vi "CRYPlot Data by Legend.vi"(4 "Flattened Scale Property":string, 5 "Frequency Symbols":i32[](array[numeric]), 6 "Flattened Plot Property":string, 7 "pGraph VI":refnum<vi>, 8 "Legend Symbols":i32[](array[numeric]), 9 "Result Rows":i32[](array[numeric]), 10 "Value Rows":i32[](array[numeric]), 11 "Rows":i32[](array[numeric])) -> ()   [LabVIEW 2013]
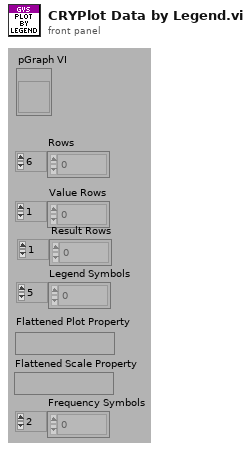
[diagram p1: front panel]
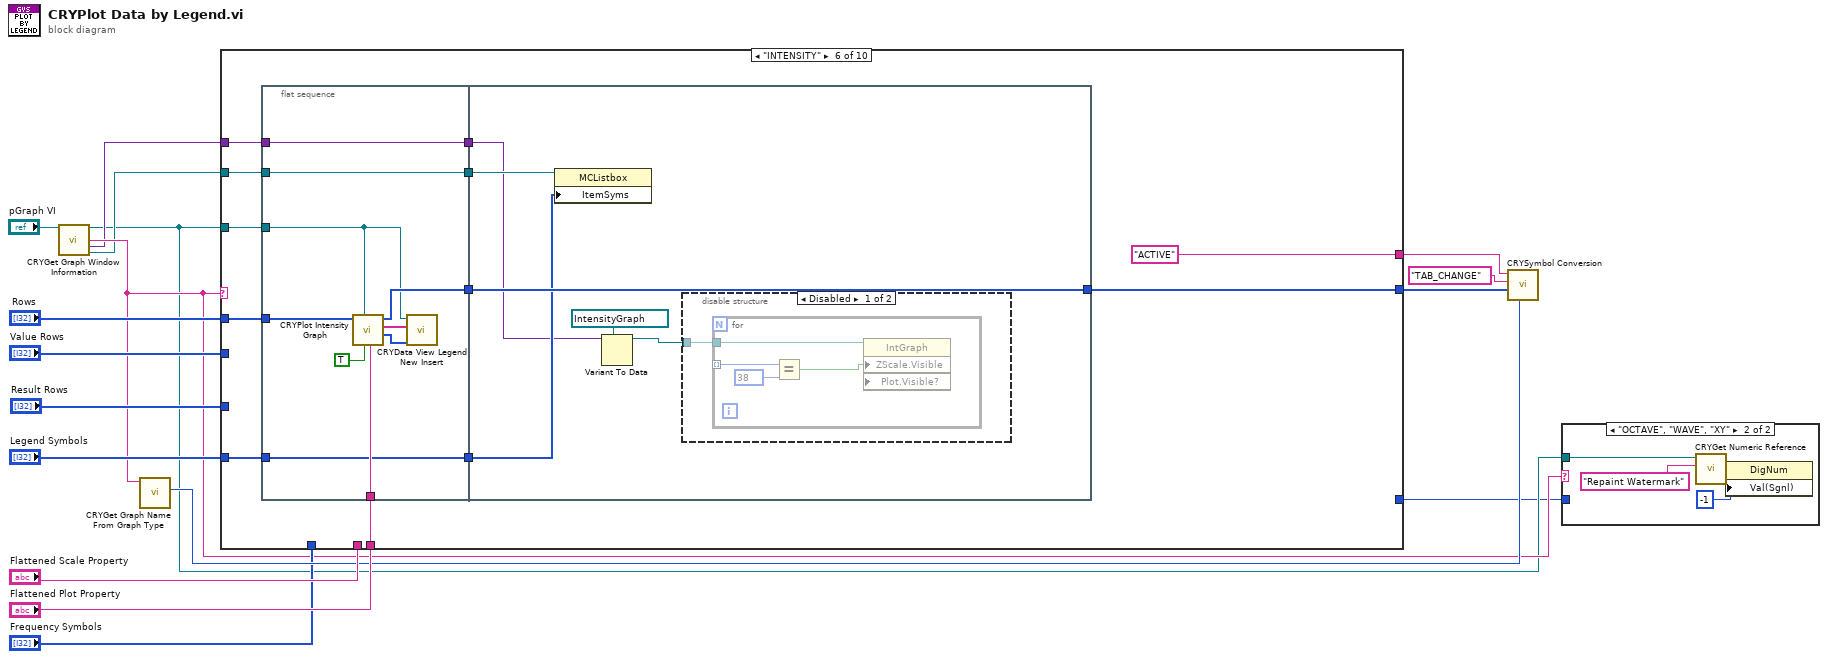
[diagram p0: block diagram]
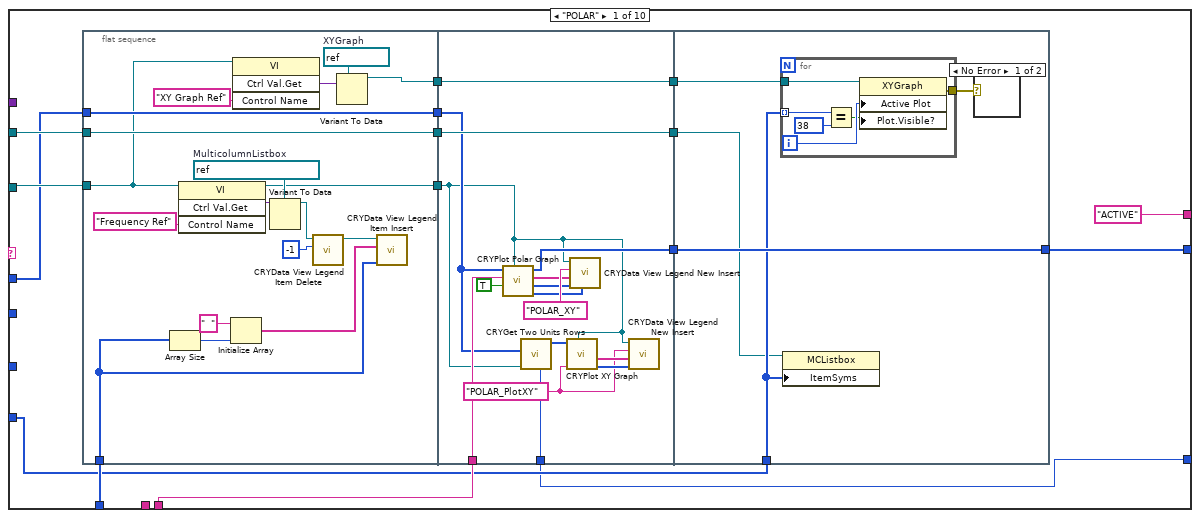
[diagram p3: hidden frame]
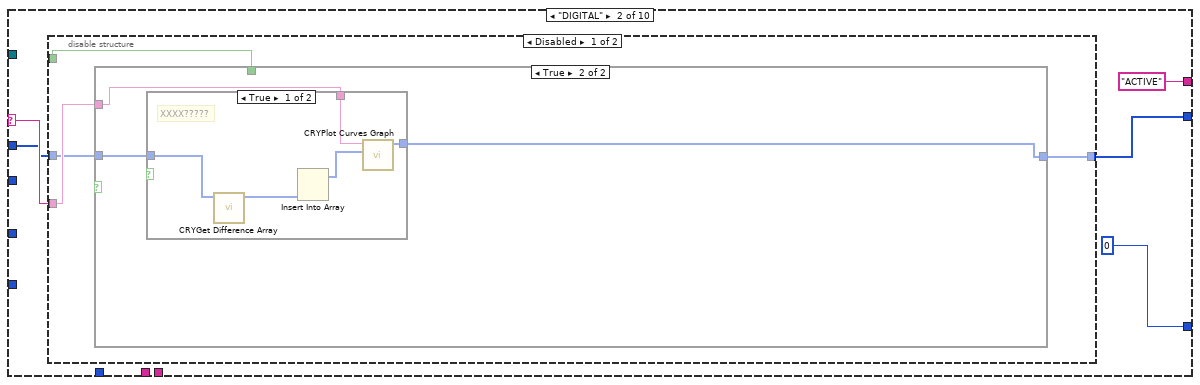
[diagram p5: hidden frame]
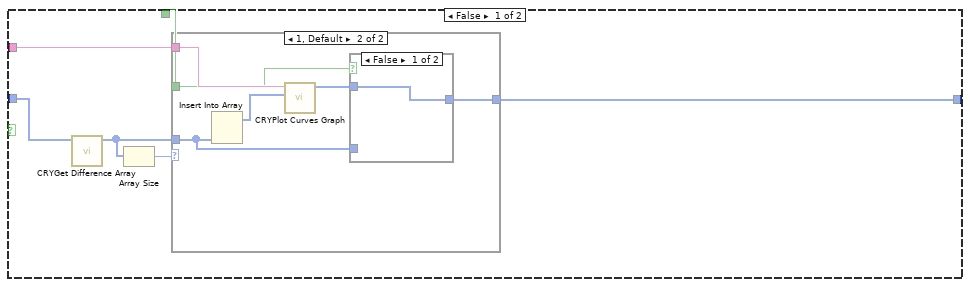
[diagram p6: hidden frame]
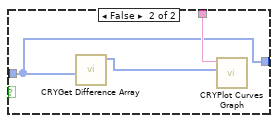
[diagram p9: hidden frame]
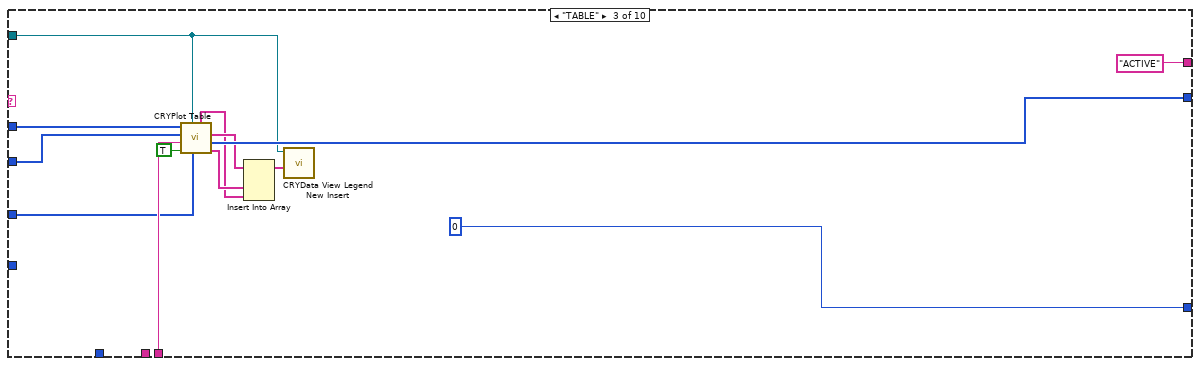
[diagram p11: hidden frame]
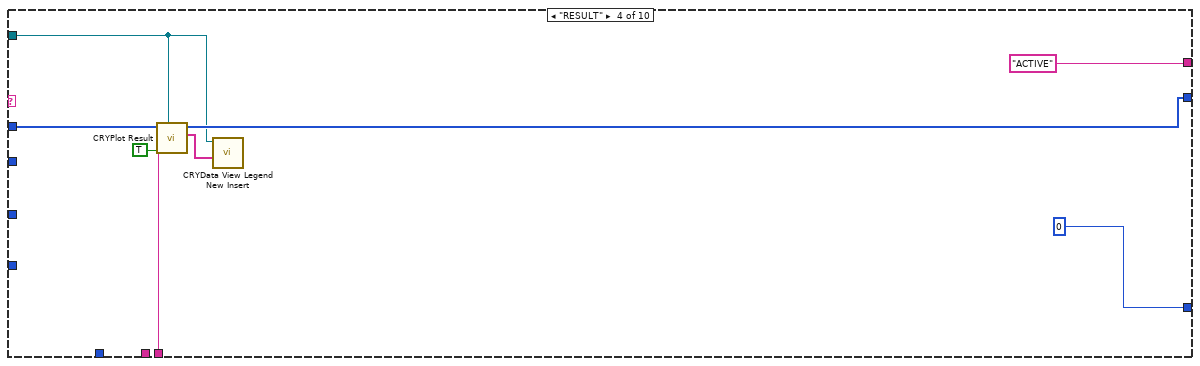
[diagram p12: hidden frame]
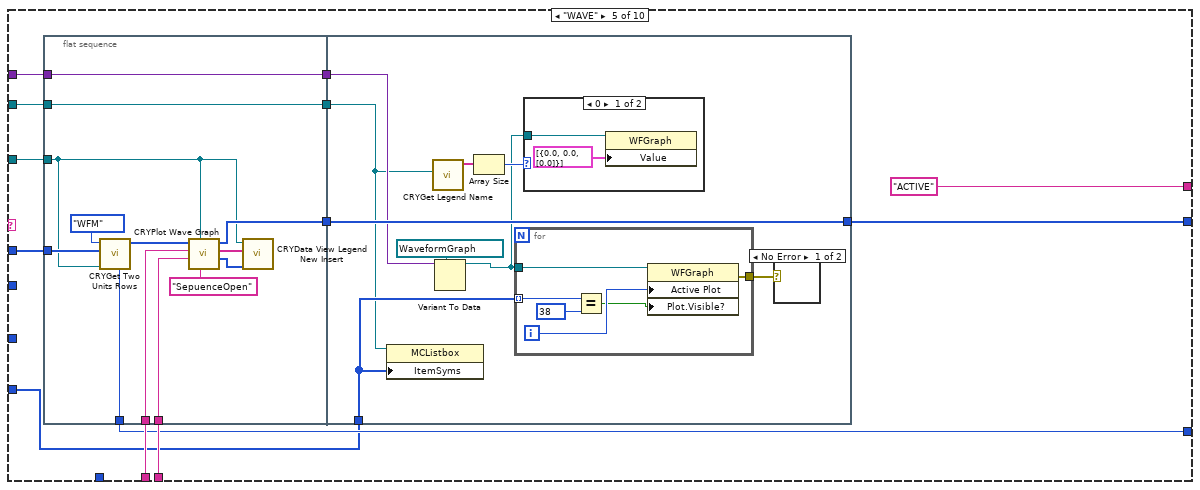
[diagram p13: hidden frame]
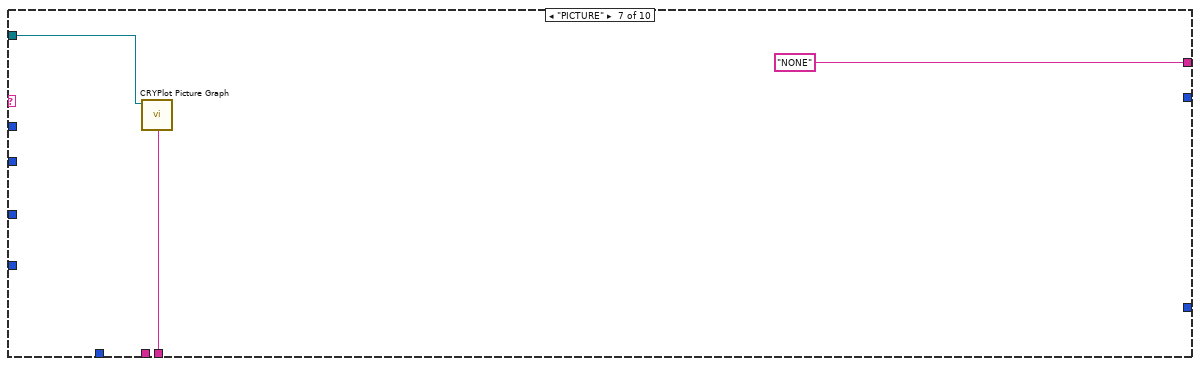
[diagram p17: hidden frame]
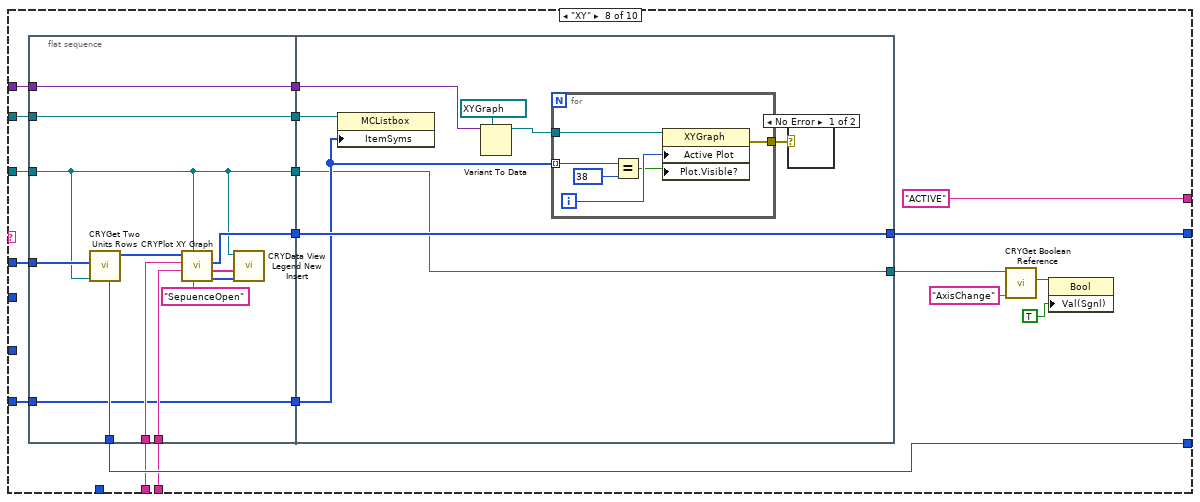
[diagram p18: hidden frame]
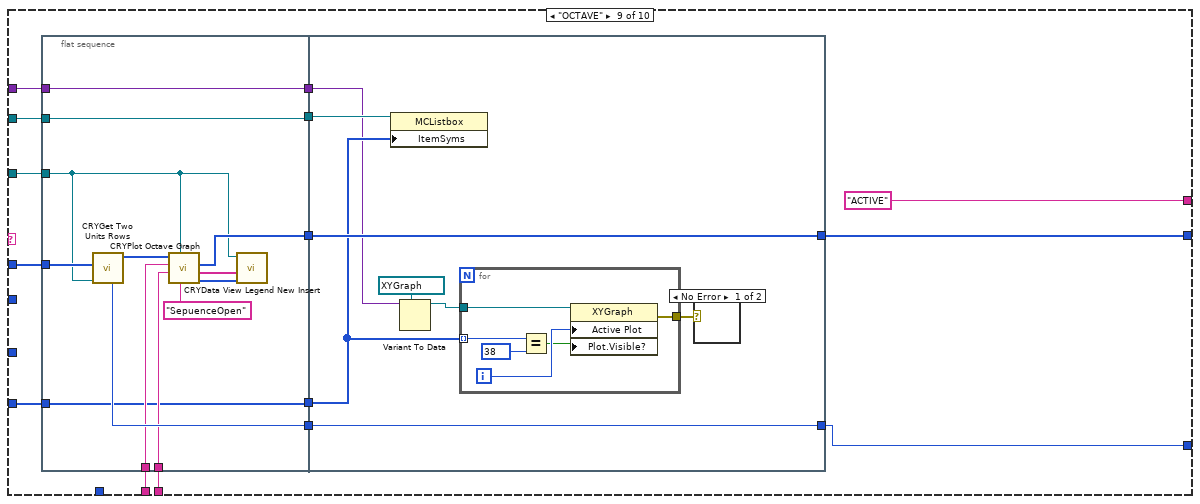
[diagram p20: hidden frame]
diagram:
  n1 = call "CRYGet Graph Window Information.vi"("pGraph VI In"="pGraph VI") -> ("pGraph VI Out"=w5:refnum<vi>, "Graph Type Out"=w9:string, "Graph Control Ref Out"=w8:variant, "Legend Ref Out"=w7:refnum<vi>)  [unwired: 4 in, 7 out]
  n2 = call "CRYGet Graph Name From Graph Type.vi"("Graph Type"=w9) -> ("Type"=w11:enum16{"Curves", "Values", "Results", "WFM"})  [unwired: 10 out]
  n3 = case shown="\"INTENSITY\"" w9 {
    selector: w9 -> [_ w83 _ _ _ _ _ _ _ _]
    tunnel: "Rows" -> [w20 w82 w121 w134 w144 w187 _ w232 w274 _]
    tunnel: [w26 0 ("Two Units") 0 ("Two Units") 0 ("Two Units") w143 _ _ w231 w273 0 ("Two Units")] -> w4
    tunnel: "Legend Symbols" -> [w27 _ _ _ w135 w185 _ w220 w266 _]
    tunnel: "Value Rows" -> [_ _ w120 _ _ _ _ _ _ _]
    tunnel: "Flattened Scale Property" -> [_ _ _ _ w146 _ _ w230 w272 _]
    tunnel: "Flattened Plot Property" -> [w31 _ w125 w132 w147 w189 w213 w229 w271 _]
    tunnel: "Result Rows" -> [_ _ w123 _ _ _ _ _ _ _]
    tunnel: [w30 w80 w122 w130 w145 w188 _ w228 w270 i32[] [] ("All Rows Out")] -> w2
    tunnel: ["ACTIVE" ("sActin") "ACTIVE" ("sActin") "ACTIVE" ("sActin") "ACTIVE" ("sActin") "ACTIVE" ("sActin") "ACTIVE" ("sActin") "NONE" ("sActin") "ACTIVE" ("sActin") "ACTIVE" ("sActin") "ACTIVE" ("sActin")] -> w1
    tunnel: w5 -> [w32 _ w114 w127 w141 w184 w211 w219 w260 _]
    tunnel: "Frequency Symbols" -> [w29 _ _ _ _ _ _ _ _ _]
    tunnel: w8 -> [_ _ _ _ w140 w178 _ w221 w267 _]
    tunnel: w7 -> [w24 _ _ _ w139 w180 _ w223 w268 _]
    frame "POLAR" {
      n4 = flat-sequence {
        tunnel: w32 -> [w40]
        tunnel: w29 -> [w34]
        tunnel: [w37] -> w25
        tunnel: w24 -> [w46]
        tunnel: [w46] -> w22
        tunnel: [w45] -> w21
        tunnel: w20 -> [w45]
        tunnel: [w41] -> w18
        tunnel: w31 -> [w63]
        tunnel: [w62] -> w28
        tunnel: [w58] -> w26
        tunnel: w25 -> [w52]
        tunnel: [w56] -> w23
        tunnel: w22 -> [w56]
        tunnel: w21 -> [w55]
        tunnel: [w54] -> w19
        tunnel: w18 -> [w54]
        tunnel: [w72] -> w30
        tunnel: w28 -> [w72]
        tunnel: w27 -> [w71]
        tunnel: w23 -> [w70]
        tunnel: w19 -> [w68]
        frame #0 {
          w42 = refnum<vi> refnum  # XYGraph
          w49 = refnum<vi> refnum  # MulticolumnListbox
          n5 = Array Size(array=w34) -> (size(s)=w47:i32)
          n6 = invoke class="VI" method="Ctrl Val.Get"(reference=w40, "Control Name"="Frequency Ref") -> (reference out=w37:refnum<vi>, "Get Control Value Variant"=w51:variant)  [unwired: 2 in, 2 out]
          n7 = Initialize Array("  ", w47) -> (w35:string[])
          n8 = invoke class="VI" method="Ctrl Val.Get"(reference=w40, "Control Name"="XY Graph Ref") -> ("Get Control Value Variant"=w43:variant)  [unwired: 2 in, 3 out]
          n9 = Variant To Data(type=w49, Variant=w51) -> (data=w36:refnum<vi>)  [unwired: 1 in, 1 out]
          n10 = call "CRYData View Legend Item Delete.vi"("RowNumber"=-1, "Legend MultiListbox In"=w36) -> ("Legend MultiListbox Out"=w39:refnum<vi>)  [unwired: 9 out]
          n11 = Variant To Data(type=w42, Variant=w43) -> (data=w41:refnum<vi>)  [unwired: 1 in, 1 out]
          n12 = call "CRYData View Legend Item Insert.vi"("Item Symbols"=w34, "ItemName Array"=w35, "Legend MultiListbox"=w39) -> ()  [unwired: 1 in, 8 out]
        }
        frame #1 {
          w53 = "POLAR_PlotXY" ("sOption")
          n13 = call "CRYPlot Polar Graph.vi"("pGraph VI In"=w52, "GraphSet"=TRUE, "Flattened Polar Property"=w63, "Selected Rows In"=w55) -> ("ItemSyms"=w57:i32[], "Freq Color"=w64:u32[], "Freq Name"=w65:string[], "Selected Row Out"=w62:i32[])  [unwired: 2 in, 2 out]
          n14 = call "CRYGet Two Units Rows.vi"("pGraph VI In"=w52, "Old Rows In"=w55) -> ("All Rows Out"=w59:i32[], "Two Units"=w58:i32)  [unwired: 3 in, 5 out]
          n15 = call "CRYPlot XY Graph.vi"("pGraph VI In"=w52, "sType"=w53, "Selected Rows In"=w59) -> ("Color Info"=w61:u32[], "Curve Name"=w60:string[])  [unwired: 3 in, 4 out]
          n16 = call "CRYData View Legend New Insert.vi"("Item Symbols"=w57, "Color Array"=w64, "ItemName Array"=w65, "sOption"="POLAR_XY", "pGraph VI In"=w52) -> ()  [unwired: 7 out]
          n17 = call "CRYData View Legend New Insert.vi"("Color Array"=w61, "ItemName Array"=w60, "sOption"=w53, "pGraph VI In"=w52) -> ()  [unwired: 1 in, 7 out]
        }
        frame #2 {
          n18 = for {
            tunnel: w71 -> [w77] mode=indexing
            tunnel: w68 -> [w74]
            tunnel: [w73] -> w69
            i -> [w76]
            n19 = Equal?(x=w77, y=38) -> (x = y?=w75:bool)
            n20 = property class="XYGraph"(reference=w74, "Active Plot"=w76, "Plot.Visible?"=w75) -> (error out=w73:errorcluster)  [unwired: 1 in, 1 out]
          }
          n21 = property on="Property Node" class="MCListbox"(reference=w70, "ItemSyms"=w71) -> ()  [unwired: 1 in, 2 out]
          n22 = case shown="No Error" w69 {
            frame No Error {
            }
            frame Error {
            }
          }
        }
      }
    }
    frame "DIGITAL" {
      n23 = disable-structure shown="Disabled" {
        disable-tunnel: w83 -> [w87 _]
        disable-tunnel: w82 -> [w86 _]
        disable-tunnel: _ -> [w85 _]
        disable-tunnel: [w84 _] -> w80
        frame Disabled {
          n24 = case shown="True" {
            selector: _ -> [_ _]
            tunnel: w87 -> [w91 w105]
            tunnel: w86 -> [w90 w104]
            tunnel: w85 -> [w89 _]
            tunnel: [w88 w103] -> w84
            frame False {
              n25 = call "CRYGet Difference Array.vi"("Array 1"=w90) -> ("Diff Out"=w93:i32[])  [unwired: 4 in, 6 out]
              n26 = Array Size(array=w93) -> (size(s)=w92:i32)
              n27 = case shown="1, Default" w92 {
                tunnel: w91 -> [_ w99]
                tunnel: w93 -> [w94 w97]
                tunnel: w89 -> [_ w96]
                tunnel: [w94 w95] -> w88
                frame 0 {
                }
                frame 1, Default {
                  n28 = Insert Into Array(new element=w97) -> (w100:i32[])  [unwired: 2 in]
                  n29 = call "CRYPlot Curves Graph.vi"("Rows In"=w100, "Graph Type"=w99) -> ("All Rows Out"=w98:i32[])  [unwired: 8 in, 1 out]
                  n30 = case shown="False" w96 {
                    tunnel: w98 -> [w101 _]
                    tunnel: w97 -> [_ w102]
                    tunnel: [w101 w102] -> w95
                    frame False {
                    }
                    frame True {
                    }
                  }
                }
              }
            }
            frame True {
              n31 = case shown="True" {
                selector: _ -> [_ _]
                tunnel: w105 -> [w109 w113]
                tunnel: w104 -> [w108 w111]
                tunnel: [w106 w111] -> w103
                frame True {
                  # "XXXX?????"
                  n32 = call "CRYGet Difference Array.vi"("Array 1"=w108) -> ("Diff Out"=w110:i32[])  [unwired: 4 in, 6 out]
                  n33 = Insert Into Array(new element=w110) -> (w107:i32[])  [unwired: 2 in]
                  n34 = call "CRYPlot Curves Graph.vi"("Rows In"=w107, "Graph Type"=w109) -> ("All Rows Out"=w106:i32[])  [unwired: 8 in, 1 out]
                }
                frame False {
                  n35 = call "CRYGet Difference Array.vi"("Array 2"=w111) -> ("Diff Out"=w112:i32[])  [unwired: 4 in, 6 out]
                  n36 = call "CRYPlot Curves Graph.vi"("Rows In"=w112, "Graph Type"=w113) -> ()  [unwired: 8 in, 2 out]
                }
              }
            }
          }
        }
        frame Enabled {
        }
      }
    }
    frame "TABLE" {
      n37 = call "CRYPlot Table.vi"("Result Rows In"=w123, "pGraph VI In"=w114, "Graph Set?"=TRUE, "Flattened Property"=w125, "Value Rows In"=w120, "Curve Rows In"=w121) -> ("Value Name"=w117:string[], "Value Rows Out"=w122:i32[], "Curve Name"=w118:string[], "Result Name"=w116:string[])  [unwired: 2 out]
      n38 = Insert Into Array(array=w118, new element #1=w117, new element #2=w116) -> (w119:string[])  [unwired: 1 in]
      n39 = call "CRYData View Legend New Insert.vi"("ItemName Array"=w119, "pGraph VI In"=w114) -> ()  [unwired: 3 in, 7 out]
    }
    frame "RESULT" {
      n40 = call "CRYPlot Result.vi"("pGraph VI In"=w127, "Graph Set?"=TRUE, "Flattened Property"=w132, "Old Rows In"=w134) -> ("Curve Name"=w129:string[], "Selected Rows Out"=w130:i32[])  [unwired: 2 in, 4 out]
      n41 = call "CRYData View Legend New Insert.vi"("ItemName Array"=w129, "pGraph VI In"=w127) -> ()  [unwired: 3 in, 7 out]
    }
    frame "WAVE" {
      n42 = flat-sequence {
        tunnel: w147 -> [w158]
        tunnel: w146 -> [w157]
        tunnel: w144 -> [w155]
        tunnel: [w154] -> w143
        tunnel: w141 -> [w148]
        tunnel: w140 -> [w150]
        tunnel: w139 -> [w149]
        tunnel: [w156] -> w138
        tunnel: [w150] -> w137
        tunnel: [w149] -> w136
        tunnel: [w169] -> w145
        tunnel: w138 -> [w169]
        tunnel: w137 -> [w165]
        tunnel: w136 -> [w161]
        tunnel: w135 -> [w166]
        frame #0 {
          n43 = call "CRYGet Two Units Rows.vi"("pGraph VI In"=w148, "Old Rows In"=w155, "Type"=enum16{"Curves", "Values", "Results", "WFM"}."WFM") -> ("All Rows Out"=w153:i32[], "Two Units"=w154:i32)  [unwired: 2 in, 5 out]
          n44 = call "CRYPlot Wave Graph.vi"("sOption"="SepuenceOpen", "pGraph VI In"=w148, "Flattened Plot Property"=w158, "Flattened Scale Property"=w157, "Selected Rows In"=w153) -> ("Color Info"=w159:u32[], "Curve Name"=w160:string[], "Selected Rows Out"=w156:i32[])  [unwired: 1 in, 3 out]
          n45 = call "CRYData View Legend New Insert.vi"("Color Array"=w159, "ItemName Array"=w160, "pGraph VI In"=w148) -> ()  [unwired: 2 in, 7 out]
        }
        frame #1 {
          n46 = property on="Property Node" class="MCListbox"(reference=w161, "ItemSyms"=w166) -> ()  [unwired: 1 in, 2 out]
          n47 = call "CRYGet Legend Name.vi"("MCListbox Refnum"=w161) -> ("Names Out"=w163:string[])  [unwired: 2 in, 8 out]
          n48 = Variant To Data(type=refnum<vi> refnum ("WaveGraph Ref"), Variant=w165) -> (data=w162:refnum<vi>)  [unwired: 1 in, 1 out]
          n49 = Array Size(array=w163) -> (size(s)=w164:i32)
          n50 = for {
            tunnel: w166 -> [w176] mode=indexing
            tunnel: w162 -> [w173]
            tunnel: [w172] -> w167
            i -> [w175]
            n51 = Equal?(x=w176, y=38) -> (x = y?=w174:bool)
            n52 = property class="WFGraph"(reference=w173, "Active Plot"=w175, "Plot.Visible?"=w174) -> (error out=w172:errorcluster)  [unwired: 1 in, 1 out]
          }
          n53 = case shown="0" w164 {
            tunnel: w162 -> [w171 _]
            frame 0 {
              n54 = property class="WFGraph"(reference=w171, "Value"=cluster{"xo":dbl, "dx":dbl, dbl[]}[] [{"xo"=0.0, "dx"=0.0, [0.0]}] ("appended array")) -> ()  [unwired: 1 in, 2 out]
            }
            frame 1, Default {
            }
          }
          n55 = case shown="No Error" w167 {
            frame No Error {
            }
            frame Error {
            }
          }
        }
      }
    }
    frame "INTENSITY" {
      n56 = flat-sequence {
        tunnel: w189 -> [w197]
        tunnel: w187 -> [w194]
        tunnel: w185 -> [w193]
        tunnel: w184 -> [w190]
        tunnel: [w195] -> w183
        tunnel: [w193] -> w182
        tunnel: [w192] -> w181
        tunnel: w180 -> [w192]
        tunnel: [w191] -> w179
        tunnel: w178 -> [w191]
        tunnel: [w205] -> w188
        tunnel: w183 -> [w205]
        tunnel: w182 -> [w204]
        tunnel: w181 -> [w202]
        tunnel: w179 -> [w201]
        frame #0 {
          n57 = call "CRYPlot Intensity Graph.vi"("Graph Set?"=TRUE, "pGraph VI In"=w190, "Flattened Intensity Property"=w197, "Selected Rows In"=w194) -> ("Color Info"=w198:u32[], "Wave Names"=w199:string[], "All Rows Out"=w195:i32[])  [unwired: 4 in, 1 out]
          n58 = call "CRYData View Legend New Insert.vi"("Color Array"=w198, "ItemName Array"=w199, "pGraph VI In"=w190) -> ()  [unwired: 2 in, 7 out]
        }
        frame #1 {
          n59 = property on="Property Node" class="MCListbox"(reference=w202, "ItemSyms"=w204) -> ()  [unwired: 1 in, 2 out]
          n60 = Variant To Data(type=refnum<vi> refnum ("Graph Ref"), Variant=w201) -> (data=w200:refnum<vi>)  [unwired: 1 in, 1 out]
          n61 = disable-structure shown="Disabled" {
            disable-tunnel: w200 -> [w206 _]
            frame Disabled {
              n62 = for {
                tunnel: _ -> [w209] mode=indexing
                tunnel: w206 -> [w208]
                n63 = Equal?(x=w209, y=38) -> (x = y?=w207:bool)
                n64 = property class="IntGraph" props=["ZScale", "Visible", "Plot", "Visible?"](reference=w208, "ZScale.Visible"=w207) -> ()  [unwired: 2 in, 2 out]
              }
            }
            frame Enabled {
            }
          }
        }
      }
    }
    frame "PICTURE" {
      n65 = call "CRYPlot Picture Graph.vi"("Flattened Property"=w213, "pGraph VI In"=w211) -> ()  [unwired: 10 in]
    }
    frame "XY" {
      n66 = flat-sequence {
        tunnel: w232 -> [w245]
        tunnel: [w244] -> w231
        tunnel: w230 -> [w240]
        tunnel: w229 -> [w239]
        tunnel: [w238] -> w226
        tunnel: [w236] -> w225
        tunnel: w220 -> [w236]
        tunnel: [w235] -> w224
        tunnel: w223 -> [w235]
        tunnel: [w234] -> w222
        tunnel: w221 -> [w234]
        tunnel: w219 -> [w233]
        tunnel: [w233] -> w218
        tunnel: [w253] -> w228
        tunnel: w226 -> [w253]
        tunnel: w225 -> [w251]
        tunnel: w224 -> [w250]
        tunnel: w222 -> [w248]
        tunnel: w218 -> [w246]
        tunnel: [w246] -> w214
        frame #0 {
          n67 = call "CRYGet Two Units Rows.vi"("pGraph VI In"=w233, "Old Rows In"=w245) -> ("All Rows Out"=w243:i32[], "Two Units"=w244:i32)  [unwired: 3 in, 5 out]
          n68 = call "CRYPlot XY Graph.vi"("sOption"="SepuenceOpen", "pGraph VI In"=w233, "Flattened Property"=w239, "Flattened Scale Property"=w240, "Selected Rows In"=w243) -> ("Color Info"=w241:u32[], "Curve Name"=w242:string[], "All Rows Out"=w238:i32[])  [unwired: 1 in, 3 out]
          n69 = call "CRYData View Legend New Insert.vi"("Color Array"=w241, "ItemName Array"=w242, "pGraph VI In"=w233) -> ()  [unwired: 2 in, 7 out]
        }
        frame #1 {
          n70 = property on="Property Node" class="MCListbox"(reference=w250, "ItemSyms"=w251) -> ()  [unwired: 1 in, 2 out]
          n71 = Variant To Data(type=refnum<vi> refnum ("XY Graph"), Variant=w248) -> (data=w247:refnum<vi>)  [unwired: 1 in, 1 out]
          n72 = for {
            tunnel: w251 -> [w258] mode=indexing
            tunnel: w247 -> [w255]
            tunnel: [w254] -> w252
            i -> [w257]
            n73 = Equal?(x=w258, y=38) -> (x = y?=w256:bool)
            n74 = property class="XYGraph"(reference=w255, "Active Plot"=w257, "Plot.Visible?"=w256) -> (error out=w254:errorcluster)  [unwired: 1 in, 1 out]
          }
          n75 = case shown="No Error" w252 {
            frame No Error {
            }
            frame Error {
            }
          }
        }
      }
      n76 = call "CRYGet Boolean Reference.vi"("Label Name"="AxisChange", "VI Refnum"=w214) -> ("Boolean Ref"=w215:refnum<vi>)  [unwired: 7 in, 2 out]
      n77 = property class="Bool"(reference=w215, "Val(Sgnl)"=TRUE) -> ()  [unwired: 1 in, 2 out]
    }
    frame "OCTAVE" {
      n78 = flat-sequence {
        tunnel: w274 -> [w287]
        tunnel: w272 -> [w282]
        tunnel: w271 -> [w281]
        tunnel: w268 -> [w278]
        tunnel: w267 -> [w277]
        tunnel: w266 -> [w276]
        tunnel: [w286] -> w265
        tunnel: [w280] -> w264
        tunnel: [w278] -> w263
        tunnel: [w277] -> w262
        tunnel: [w276] -> w261
        tunnel: w260 -> [w275]
        tunnel: [w294] -> w270
        tunnel: [w295] -> w273
        tunnel: w265 -> [w295]
        tunnel: w264 -> [w294]
        tunnel: w263 -> [w293]
        tunnel: w262 -> [w288]
        tunnel: w261 -> [w292]
        frame #0 {
          n79 = call "CRYGet Two Units Rows.vi"("pGraph VI In"=w275, "Old Rows In"=w287) -> ("All Rows Out"=w285:i32[], "Two Units"=w286:i32)  [unwired: 3 in, 5 out]
          n80 = call "CRYPlot Octave Graph.vi"("sOption"="SepuenceOpen", "pGraph VI In"=w275, "Flattened Property"=w281, "Flattened Scale Property"=w282, "Selected Rows In"=w285) -> ("Color Info"=w283:u32[], "Curve Name"=w284:string[], "All Rows Out"=w280:i32[])  [unwired: 3 in, 1 out]
          n81 = call "CRYData View Legend New Insert.vi"("Color Array"=w283, "ItemName Array"=w284, "pGraph VI In"=w275) -> ()  [unwired: 2 in, 7 out]
        }
        frame #1 {
          n82 = property on="Property Node" class="MCListbox"(reference=w293, "ItemSyms"=w292) -> ()  [unwired: 1 in, 2 out]
          n83 = Variant To Data(type=refnum<vi> refnum ("WaveGraph Ref"), Variant=w288) -> (data=w289:refnum<vi>)  [unwired: 1 in, 1 out]
          n84 = for {
            tunnel: w292 -> [w300] mode=indexing
            tunnel: w289 -> [w297]
            tunnel: [w296] -> w291
            i -> [w299]
            n85 = Equal?(x=w300, y=38) -> (x = y?=w298:bool)
            n86 = property class="XYGraph"(reference=w297, "Active Plot"=w299, "Plot.Visible?"=w298) -> (error out=w296:errorcluster)  [unwired: 1 in, 1 out]
          }
          n87 = case shown="No Error" w291 {
            frame No Error {
            }
            frame Error {
            }
          }
        }
      }
    }
    frame Default {
    }
  }
  n88 = call "CRYSymbol Conversion.vi"("CurLib Tab Type"=w11, "nDatas"=w2, "sData"="TAB_CHANGE" ("sActin"), "sActin"=w1) -> ()  [unwired: 8 in]
  n89 = case shown="\"OCTAVE\", \"WAVE\", \"XY\"" w9 {
    tunnel: w5 -> [_ w306]
    tunnel: w4 -> [_ _]
    frame Default {
    }
    frame "OCTAVE", "WAVE", "XY" {
      n90 = call "CRYGet Numeric Reference.vi"("Label Name"="Repaint Watermark" ("Control Name"), "VI Refnum"=w306) -> ("Numeric Ref Out"=w308:refnum<vi>)  [unwired: 9 out]
      n91 = property class="DigNum"(reference=w308, "Val(Sgnl)"=-1 ("Two Units")) -> ()  [unwired: 1 in, 2 out]
    }
  }
